vi "Start_XNETSesion.vi"(3 "error in (no error)":errorcluster, 6 "Model":string) -> (0 "error out":errorcluster, 1 "Read":refnum<k21>, 2 "Write":refnum<k21>)   [LabVIEW 2023]
uses:
  <vilib>/xnet/xnet.llb/XNET Create Session (Frame Input Stream).vi
  <vilib>/xnet/xnet.llb/XNET Create Session (Frame Output Queued).vi
  <resource>/objmgr/xnet.rc
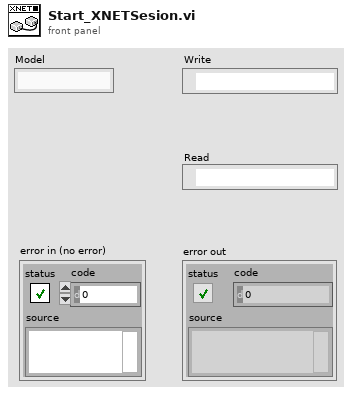
[diagram p1: front panel]
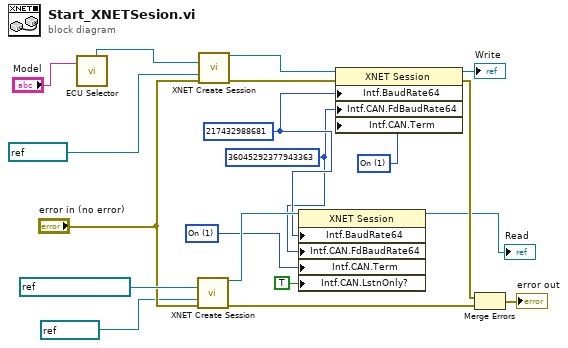
[diagram p0: block diagram]
diagram:
  w7 = u32 1 items=["Off", "On"] ("Interface:CAN:Termination")
  w17 = u32 1 items=["Off", "On"] ("Interface:CAN:Termination")
  w8 = u64 36045292377943363 ("Interface:CAN:64bit FD Baud Rate")
  w9 = u64 217432988681 ("Interface:64bit Baud Rate")
  n1 = call "ECU Selector.vi"("Model"="Model") -> ("frame"=w1:refnum<k21>)  [unwired: 1 in, 4 out]
  n2 = call-poly <vilib>:"XNET Create Session.vi"("cluster (:memory:)"=refnum<k21> "Elatch Database", "interface"=refnum<k21> "CAN2", "error in (no error)"="error in (no error)") -> ("session out"=w10:refnum<k21>, "error out"=w13:errorcluster)  [unwired: 11 in]
  n3 = call-poly <vilib>:"XNET Create Session.vi"("frame"=w1, "interface"=refnum<k21> "CAN1", "error in (no error)"="error in (no error)") -> ("session out"=w16:refnum<k21>, "error out"=w19:errorcluster)  [unwired: 11 in]
  n4 = property class="XNET Session"(reference=w10, "Intf.BaudRate64"=w9, "Intf.CAN.FdBaudRate64"=w8, "Intf.CAN.Term"=w7, "Intf.CAN.LstnOnly?"=TRUE ("Interface:CAN:Listen Only?")) -> (reference out=→"Read":refnum<k21>)  [unwired: 1 in, 1 out]
  n5 = property class="XNET Session"(reference=w16, error in=w19, "Intf.BaudRate64"=w9, "Intf.CAN.FdBaudRate64"=w8, "Intf.CAN.Term"=w17) -> (reference out=→"Write":refnum<k21>, error out=w12:errorcluster)
  n6 = Merge Errors(w12, w13) -> (→"error out":errorcluster)
